vi "pco.camera_SaveImages_Example.vi"() -> ()   [LabVIEW 2019]
uses:
  pco.camera/Camera.lvclass
  pco.recorder/Recorder.lvlib
  <vilib>/picture/picture.llb/Draw 8-Bit Pixmap.vi
  <vilib>/picture/picture.llb/Draw True-Color Pixmap.vi
panel:
  out "colormap(U8)":u32[](array[numeric])
  out "Image(U16)":u16[][](graph)
  in  "Zoom [%]":i32(c297)=26
  out "Image":picture
  out "rawImage":u16[][](array[numeric])
  in  "data_format":T1(ring)=enum."Mono16"
  in  "Image Index":u32 max=9
  in  "saveImages":bool
  in  "SavePath":path
  out "Recorded Images":u32
  in  "Quit":bool
  in  "roiY1":u64=2 min=2 max=5120 step=1
  in  "roiX1":u64=2 min=2 max=5120 step=1
  in  "roiY0":u64=1 min=1 max=5119 step=1
  in  "roiX0":u64=1 min=1 max=5119 step=1
  out "Image Height":u16
  out "Image Width":u16
  in  "dwImgCount":u32=10 caption="Required Number of Images" max=4023
  out "Error":errorcluster {"code" format="%x"}
  # "This example shows how to record an image sequence and save all images to files (and an .avi) afterwards.\nIt is a good starting point for writing own applications with file saving\nBut it will not be fail save, i.e. doesnt react on errors, just handles them forward to the end\n\nUsage:\nSelect your required image count you want to record before you start the program.\nOnce started, the camera class will be initialized and images will be recorded automatically.\nWhen acquisition has finished you can read the images by index, crop them using the ROI parameters and select a file path.\nBy clicking save, the images are saved with the selected file format using the current active roi setting.\nThis also finishes the program and will force an exit of the camera class"
  # "pco.labview"
  # "Camera Setup"
  # "Recording Control"
  # "Parameters for image readout"
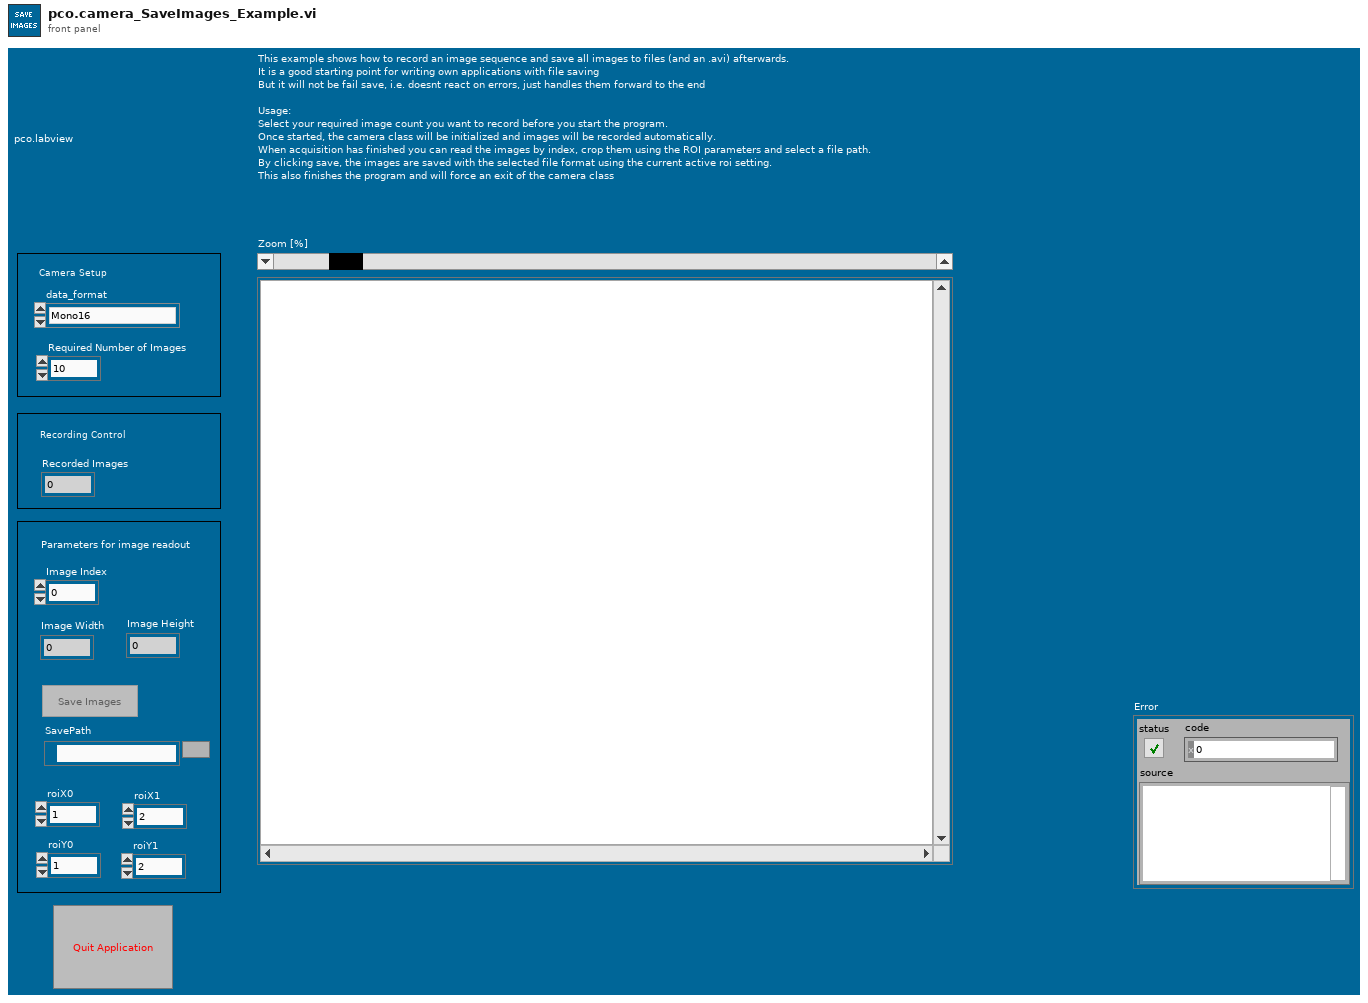
[diagram p1: front panel]
types:
  T1 = enum16{"Undefined", "Mono8", "Mono16", "BGRA8", "RGBA8", "BGRA16", "RGBA16", "CompressedMono8"}
  T2 = enum8{"Enabled", "Disabled", "Disabled and Grayed Out"}
  T3 = enum16{"sequence", "sequence non blocking", "ring buffer", "fifo", "sequence_dpcore", "sequence_non_blocking_dpcore", "ring_buffer_dpcore", "fifo_dpcore", "tif", "multitif", "pcoraw", "b16", "dicom", "multidicom"}
  T4 = typedef "Camera.lvclass/binning.ctl" = cluster{"vert":u16, "horz":u16}
  T5 = cluster{"exposure_time_s":dbl, "delay_time_s":dbl, "roi":cluster{"x0":u64, "y0":u64, "x1":u64, "y1":u64}, "timestamp_mode":u16, "pixelrate":u32, "trigger_mode":u16, "acquire_mode":u16, "metadata_mode":u16, "noisefilter_mode":u16, "binning":T4}
  T6 = cluster{"wVersion":u16, "dwIMAGE_COUNTER":u32, "dwIMAGE_TIME_US":u32, "lvTimestamp":timestamp, "bIMAGE_TIME_STATUS":u8, "wEXPOSURE_TIME_BASE":u16, "dwEXPOSURE_TIME":u32, "dwFRAMERATE_MILLIHZ":u32, "sSENSOR_TEMPERATURE":i16, "wIMAGE_SIZE_X":u16, "wIMAGE_SIZE_Y":u16, "bBINNING_X":u8, "bBINNING_Y":u8, "dwSENSOR_READOUT_FREQUENCY":u32, "wSENSOR_CONV_FACTOR":u16, "dwCAMERA_SERIAL_NO":u32, "wCAMERA_TYPE":u16, "bBIT_RESOLUTION":u8, "bSYNC_STATUS":u8, "wDARK_OFFSET":u16, "bTRIGGER_MODE":u8, "bDOUBLE_IMAGE_MODE":u8, "bCAMERA_SYNC_MODE":u8, "bIMAGE_TYPE":u8, "wCOLOR_PATTERN":u16, "wCAMERA_SUBTYPE":u16, "dwEVENT_NUMBER":u32, "wIMAGE_SIZE_X_Offset":u16, "wIMAGE_SIZE_Y_Offset":u16}[]
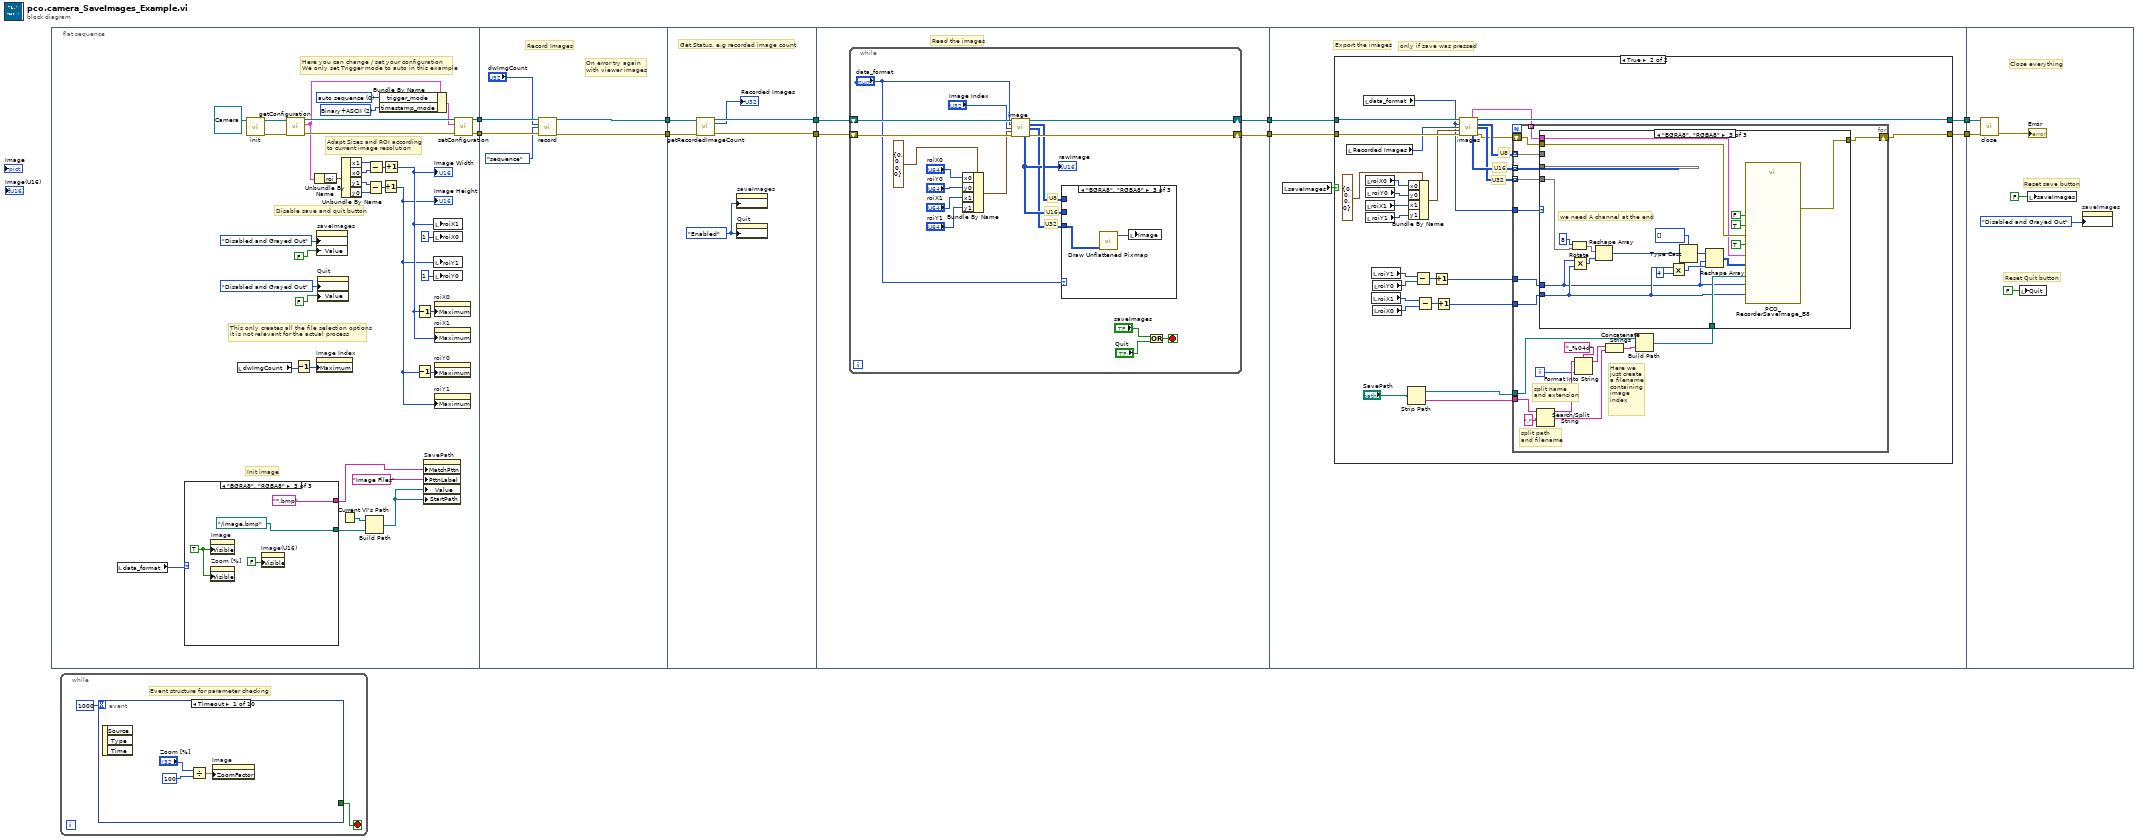
[diagram p0: block diagram]
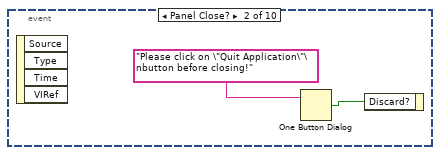
[diagram p2: hidden frame]
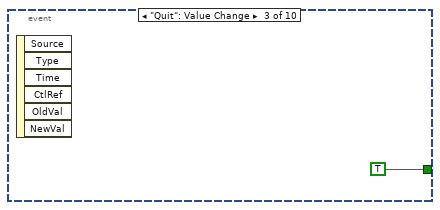
[diagram p3: hidden frame]
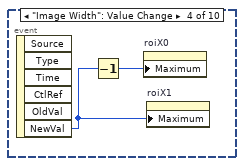
[diagram p4: hidden frame]
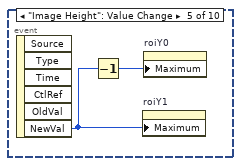
[diagram p5: hidden frame]
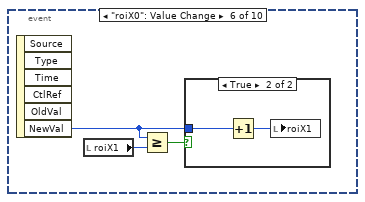
[diagram p6: hidden frame]
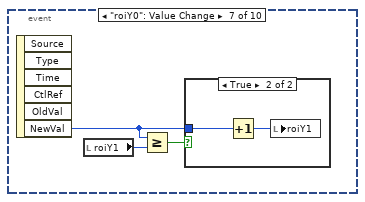
[diagram p8: hidden frame]
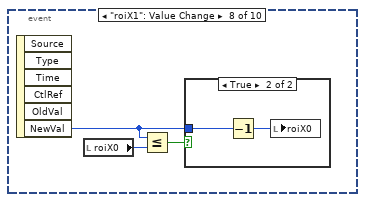
[diagram p10: hidden frame]
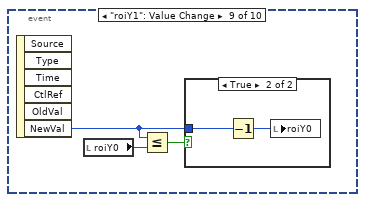
[diagram p12: hidden frame]
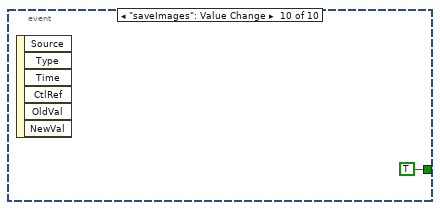
[diagram p14: hidden frame]
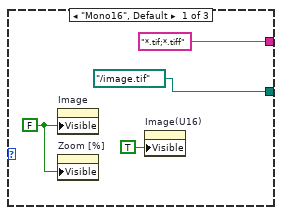
[diagram p15: hidden frame]
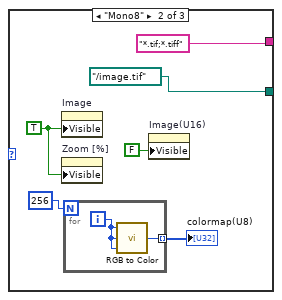
[diagram p16: hidden frame]
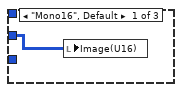
[diagram p17: hidden frame]
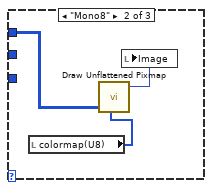
[diagram p18: hidden frame]
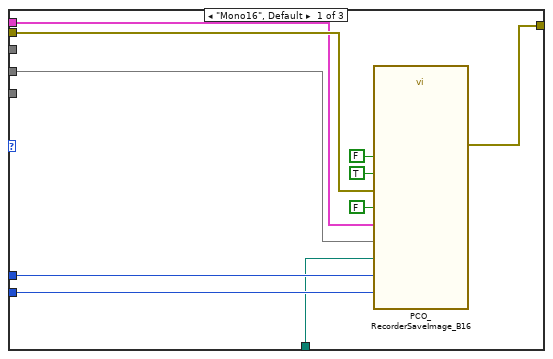
[diagram p20: hidden frame]
diagram:
  n1 = flat-sequence {
    tunnel: [w37] -> w10
    tunnel: [w36] -> w9
    tunnel: w10 -> [w68]
    tunnel: w9 -> [w67]
    tunnel: [w65] -> w8
    tunnel: [w64] -> w7
    tunnel: w8 -> [w74]
    tunnel: w7 -> [w73]
    tunnel: [w72] -> w6
    tunnel: [w71] -> w5
    tunnel: w6 -> [w77]
    tunnel: w5 -> [w78]
    tunnel: [w76] -> w4
    tunnel: [w75] -> w2
    tunnel: w4 -> [w106]
    tunnel: [w105] -> w3
    tunnel: w2 -> [w104]
    tunnel: [w103] -> w1
    tunnel: w3 -> [w201]
    tunnel: w1 -> [w200]
    frame #0 {
      w21 = u16 2 items=["OFF", "Binary", "Binary+ASCII", "ASCII"] ("TimestampMode")
      w43 = u16 0 items=["auto sequence"=0, "software trigger"=1, "external exposure start & software trigger"=2, "external exposure control"=3, "external synchronized"=4, "fast external exposure control"=5, "external CDS control"=6, "slow external exposure control"=7, "external synchronized HDSDI"=258] ("TriggerMode")
      # "Init image"
      # "This only creates all the file selection options\nit is not relevant for the actual process"
      # "Adapt Sizes and ROI according\nto current image resolution"
      # "Disable save and quit button"
      # "Here you can change / set your configuration\nWe only set Trigger mode to auto in this example"
      n2 = local read "data_format"() -> (w13:T1)
      n3 = case shown="\"BGRA8\", \"RGBA8\"" w13 {
        tunnel: [path "../image.tif" ("SavePath") path "../image.tif" ("SavePath") path "../image.bmp" ("SavePath")] -> w12
        tunnel: ["*.tif;*.tiff" ("pattern (all files)") "*.tif;*.tiff" ("pattern (all files)") "*.bmp" ("pattern (all files)")] -> w11
        frame "Mono16", Default {
          w49 = FALSE ("Visible")
          n4 = property on="Image" class="Pict"("Visible"=w49) -> ()  [unwired: 2 in, 2 out]
          n5 = property on="Zoom [%]" class="Scroll (strict)"("Visible"=w49) -> ()  [unwired: 2 in, 2 out]
          n6 = property on="Image(U16)" class="IntGraph (strict)"("Visible"=TRUE) -> ()  [unwired: 2 in, 2 out]
        }
        frame "Mono8" {
          w55 = TRUE ("Visible")
          n7 = property on="Image" class="Pict"("Visible"=w55) -> ()  [unwired: 2 in, 2 out]
          n8 = property on="Zoom [%]" class="Scroll (strict)"("Visible"=w55) -> ()  [unwired: 2 in, 2 out]
          n9 = for {
            N: 256 -> [_]
            tunnel: [w57] -> w54 mode=indexing
            i -> [w58]
            n10 = call <vilib>:"RGB to Color.vi"("B"=w58, "G"=w58, "R"=w58) -> ("Color"=w57:u32)
          }
          "colormap(U8)" <- w54
          n11 = property on="Image(U16)" class="IntGraph (strict)"("Visible"=FALSE) -> ()  [unwired: 2 in, 2 out]
        }
        frame "BGRA8", "RGBA8" {
          w61 = TRUE ("Visible")
          n12 = property on="Image" class="Pict"("Visible"=w61) -> ()  [unwired: 2 in, 2 out]
          n13 = property on="Zoom [%]" class="Scroll (strict)"("Visible"=w61) -> ()  [unwired: 2 in, 2 out]
          n14 = property on="Image(U16)" class="IntGraph (strict)"("Visible"=FALSE) -> ()  [unwired: 2 in, 2 out]
        }
      }
      n15 = local read "dwImgCount"() -> (w14:u32)
      n16 = call-dynamic "init.vi"("Camera in"=refnum<class "Camera.lvclass"> refnum ("PCOCamera in")) -> ("Camera out"=w45:refnum<class "Camera.lvclass">, "error out"=w44:errorcluster)  [unwired: 8 in]
      n17 = call-dynamic "getConfiguration.vi"("error in (no error)"=w44, "Camera in"=w45) -> ("error out"=w41:errorcluster, "configuration"=w31:T5, "Camera out"=w42:refnum<class "Camera.lvclass">)  [unwired: 7 in]
      n18 = Decrement(x=w14) -> (x-1=w15:u32)
      n19 = Unbundle By Name(w31) -> ("roi"=w30:cluster{"x0":u64, "y0":u64, "x1":u64, "y1":u64})
      n20 = property on="Image Index" class="DigNum (strict)"("Maximum"=w15) -> ()  [unwired: 2 in, 2 out]
      n21 = property on="saveImages" class="Bool (strict)"("DisabledEnum"=T2."Disabled and Grayed Out" ("Disabled"), "Value"=FALSE ("Stop")) -> ()  [unwired: 2 in, 2 out]
      n22 = property on="Quit" class="Bool (strict)"("DisabledEnum"=T2."Disabled and Grayed Out" ("Disabled"), "Value"=FALSE ("Stop")) -> ()  [unwired: 2 in, 2 out]
      n23 = Current VI's Path() -> (path=w18:path)
      n24 = Unbundle By Name(w30) -> ("x1"=w28:u64, "x0"=w29:u64, "y1"=w26:u64, "y0"=w27:u64)
      n25 = Build Path(base path=w18, name or relative path=w12) -> (appended path=w16:path)
      n26 = Subtract(x=w26, y=w27) -> (x-y=w24:u64)
      n27 = Subtract(x=w28, y=w29) -> (x-y=w25:u64)
      n28 = Bundle By Name(cluster=w31, "trigger_mode"=w43, "timestamp_mode"=w21) -> (w40:T5)
      n29 = Increment(x=w24) -> (x+1=w22:u64)
      "Image Height" <- w22
      n30 = Increment(x=w25) -> (x+1=w23:u64)
      "Image Width" <- w23
      n31 = Decrement(x=w23) -> (x-1=w33:u64)
      n32 = Decrement(x=w22) -> (x-1=w32:u64)
      n33 = property on="SavePath" class="Path"("MatchPttn"=w11, "PttnLabel"="Image Files" ("pattern label"), "Value"=w16, "StartPath"=w16) -> ()  [unwired: 2 in, 2 out]
      n34 = local write "roiX1"(w23) -> ()
      n35 = local write "roiX0"(u16 1 ("roiY0")) -> ()
      n36 = local write "roiY1"(w22) -> ()
      n37 = local write "roiY0"(u16 1 ("roiY0")) -> ()
      n38 = property on="roiX0" class="DigNum (strict)"("Maximum"=w33) -> ()  [unwired: 2 in, 2 out]
      n39 = property on="roiX1" class="DigNum (strict)"("Maximum"=w23) -> ()  [unwired: 2 in, 2 out]
      n40 = property on="roiY0" class="DigNum (strict)"("Maximum"=w32) -> ()  [unwired: 2 in, 2 out]
      n41 = property on="roiY1" class="DigNum (strict)"("Maximum"=w22) -> ()  [unwired: 2 in, 2 out]
      n42 = call-dynamic "setConfiguration.vi"("error in (no error)"=w41, "configuration"=w40, "Camera in"=w42) -> ("error out"=w36:errorcluster, "Camera out"=w37:refnum<class "Camera.lvclass">)  [unwired: 7 in]
    }
    frame #1 {
      # "On error try again \nwith viewer images"
      # "Record Images"
      n43 = call-dynamic "record.vi"("Camera in"=w68, "num_images"="dwImgCount", "record_mode"=T3."sequence", "error in (no error)"=w67) -> ("Camera out"=w65:refnum<class "Camera.lvclass">, "error out"=w64:errorcluster)  [unwired: 10 in]
    }
    frame #2 {
      w69 = T2."Enabled" ("Disabled")
      # "Get Status, e.g recorded image count"
      n44 = call-dynamic "getRecordedImageCount.vi"("Camera in"=w74, "error in (no error)"=w73) -> ("Camera out"=w72:refnum<class "Camera.lvclass">, "recorded_image_count"=→"Recorded Images":u32, "error out"=w71:errorcluster)  [unwired: 11 in]
      n45 = property on="saveImages" class="Bool (strict)"("DisabledEnum"=w69) -> ()  [unwired: 2 in, 2 out]
      n46 = property on="Quit" class="Bool (strict)"("DisabledEnum"=w69) -> ()  [unwired: 2 in, 2 out]
    }
    frame #3 {
      # "Read the images"
      n47 = while {
        shift-right: [w94] -> w76
        shift-left: w77 -> [w96]
        shift-right: [w89] -> w75
        shift-left: w78 -> [w95]
        stop <- w87 stop-if-true
        # "U32"
        # "U16"
        # "U8"
        n48 = Bundle By Name(cluster=cluster{"x0":u64, "y0":u64, "x1":u64, "y1":u64} {"x0"=0, "y0"=0, "x1"=0, "y1"=0} ("roi"), "x0"="roiX0", "y0"="roiY0", "x1"="roiX1", "y1"="roiY1") -> (w85:cluster{"x0":u64, "y0":u64, "x1":u64, "y1":u64})
        n49 = call-dynamic "image.vi"("Camera in"=w96, "data_format"="data_format", "image_index"="Image Index", "roi"=w85, "error in (no error)"=w95) -> ("Camera out"=w94:refnum<class "Camera.lvclass">, "image (U8)"=w82:u8[][], "image (U32)"=w80:u32[][], "raw_image (U16)"=w81:u16[][], "error out"=w89:errorcluster)  [unwired: 3 in, 3 out]
        "rawImage" <- w81
        n50 = case shown="\"BGRA8\", \"RGBA8\"" "data_format" {
          tunnel: w80 -> [_ _ w102]
          tunnel: w82 -> [_ w100 _]
          tunnel: w81 -> [w97 _ _]
          frame "Mono16", Default {
            n51 = local write "Image(U16)"(w97) -> ()
          }
          frame "Mono8" {
            n52 = local read "colormap(U8)"() -> (w99:u32[])
            n53 = call-poly <vilib>:"Draw Unflattened Pixmap.vi"("data"=w100, "color table"=w99) -> ("new picture"=w98:picture)  [unwired: 7 in]
            n54 = local write "Image"(w98) -> ()
          }
          frame "BGRA8", "RGBA8" {
            n55 = call-poly <vilib>:"Draw Unflattened Pixmap.vi"("data (RGB format)"=w102) -> ("new picture"=w101:picture)  [unwired: 8 in]
            n56 = local write "Image"(w101) -> ()
          }
        }
        n57 = Or(x="saveImages", y="Quit") -> (x .or. y?=w87:bool)
      }
    }
    frame #4 {
      # "only if save was pressed"
      # "Export the images"
      n58 = local read "saveImages"() -> (w107:bool)
      n59 = case shown="True" w107 {
        tunnel: w106 -> [w109 w136]
        tunnel: [w109 w125] -> w105
        tunnel: w104 -> [w108 w137]
        tunnel: [w108 w119] -> w103
        frame False {
        }
        frame True {
          # "U32"
          # "U16"
          # "U8"
          n60 = local read "Recorded Images"() -> (w129:u32)
          n61 = local read "data_format"() -> (w124:T1)
          n62 = local read "roiX0"() -> (w134:u64)
          n63 = local read "roiX1"() -> (w132:u64)
          n64 = local read "roiY0"() -> (w133:u64)
          n65 = local read "roiY1"() -> (w131:u64)
          n66 = local read "roiY1"() -> (w116:u64)
          n67 = local read "roiX1"() -> (w114:u64)
          n68 = local read "roiY0"() -> (w115:u64)
          n69 = local read "roiX0"() -> (w113:u64)
          n70 = Strip Path(path="SavePath") -> (stripped path=w121:path, name=w122:string)
          n71 = Bundle By Name(cluster=cluster{"x0":u64, "y0":u64, "x1":u64, "y1":u64} {"x0"=0, "y0"=0, "x1"=0, "y1"=0} ("roi"), "x0"=w134, "y0"=w133, "x1"=w132, "y1"=w131) -> (w130:cluster{"x0":u64, "y0":u64, "x1":u64, "y1":u64})
          n72 = Subtract(x=w116, y=w115) -> (x-y=w118:u64)
          n73 = Subtract(x=w114, y=w113) -> (x-y=w117:u64)
          n74 = Increment(x=w118) -> (x+1=w111:u64)
          n75 = Increment(x=w117) -> (x+1=w112:u64)
          n76 = call-dynamic "images.vi"("Camera in"=w136, "data_format"=w124, "image_count"=w129, "roi"=w130, "error in (no error)"=w137) -> ("meta_data_list"=w110:T6, "Camera out"=w125:refnum<class "Camera.lvclass">, "image_list (U8)"=w128:u8[][][], "image_list (U32)"=w126:u32[][][], "raw_image_list (U16)"=w127:u16[][][], "error out"=w120:errorcluster)  [unwired: 3 in, 2 out]
          n77 = for {
            tunnel: w128 -> [w156] mode=indexing
            tunnel: w127 -> [w155] mode=indexing
            tunnel: w126 -> [w139] mode=indexing
            tunnel: w124 -> [w147]
            tunnel: w122 -> [w146]
            tunnel: w121 -> [w145]
            shift-right: [w143] -> w119
            shift-left: w120 -> [w144]
            tunnel: w112 -> [w140]
            tunnel: w111 -> [w141]
            tunnel: w110 -> [w142] mode=indexing
            i -> [w148]
            # "Here we \njust create\na filename\ncontaining\nimage \nindex"
            # "split path \nand filename"
            # "split name \nand extension"
            n78 = Search/Split String(string=w146, search string/char (-)=".") -> (substring before match=w152:string, match + rest of string=w153:string)  [unwired: 1 in, 1 out]
            n79 = Format Into String(format string="_%04d", initial string=w152, w148) -> (resulting string=w154:string)  [unwired: 1 in, 1 out]
            n80 = Concatenate Strings(w154, w153) -> (w149:string)
            n81 = Build Path(base path=w145, name or relative path=w149) -> (appended path=w138:path)
            n82 = case shown="\"BGRA8\", \"RGBA8\"" w147 {
              tunnel: w156 -> [_ w173 _]
              tunnel: w155 -> [w161 _ _]
              tunnel: w141 -> [w163 w171 w180]
              tunnel: w140 -> [w162 w170 w181]
              tunnel: w144 -> [w160 w172 w192]
              tunnel: [w159 w169 w191] -> w143
              tunnel: w142 -> [w158 w168 w190]
              tunnel: w139 -> [_ _ w178]
              tunnel: w138 -> [w157 w167 w189]
              frame "Mono16", Default {
                n83 = call "PCO_RecorderSaveImage_B16.vi"("pImgBuf"=w161, "wWidth"=w162, "wHeight"=w163, "szFilePath"=w157, "error in (no error)"=w160, "isColor"=FALSE, "bIsBitmap"=FALSE, "PCO_METADATA_STRUCT"=w158, "bOverwrite"=TRUE) -> ("error out"=w159:errorcluster)  [unwired: 9 in, 1 out]
              }
              frame "Mono8" {
                n84 = call "PCO_RecorderSaveImage_B8.vi"("pImgBuf"=w173, "wWidth"=w170, "wHeight"=w171, "szFilePath"=w167, "error in (no error)"=w172, "isColor"=FALSE, "bIsBitmap"=FALSE, "PCO_METADATA_STRUCT"=w168, "bOverwrite"=TRUE) -> ("error out"=w169:errorcluster)  [unwired: 9 in, 1 out]
              }
              frame "BGRA8", "RGBA8" {
                # "we need A channel at the end"
                n85 = Rotate(1:w178, 2:i16 8 ("y")) -> (0:w177:u32[][])
                n86 = Multiply(x=w180, y=w181) -> (x*y=w183:u64)
                n87 = Reshape Array(w177, w183) -> (w182:u32[])
                n88 = Multiply(x=w181, y=u64 4) -> (x*y=w187:u64)
                n89 = Type Cast(type=u8[] [] ("image_list (U32)"), x=w182) -> (*(type *) &x=w188:u8[])
                n90 = Reshape Array(w188, w180, w187) -> (w184:u8[][])
                n91 = call "PCO_RecorderSaveImage_B8.vi"("pImgBuf"=w184, "wWidth"=w181, "wHeight"=w180, "szFilePath"=w189, "error in (no error)"=w192, "isColor"=TRUE, "bIsBitmap"=FALSE, "PCO_METADATA_STRUCT"=w190, "bOverwrite"=TRUE) -> ("error out"=w191:errorcluster)  [unwired: 9 in, 1 out]
              }
            }
          }
        }
      }
    }
    frame #5 {
      # "Reset Quit button"
      # "Close everything"
      # "Reset save button"
      n92 = call-dynamic "close.vi"("error in (no error)"=w200, "Camera in"=w201) -> ("error out"=→"Error":errorcluster)  [unwired: 9 in]
      n93 = local write "Quit"(FALSE ("Stop")) -> ()
      n94 = local write "saveImages"(FALSE ("Stop")) -> ()
      n95 = property on="saveImages" class="Bool (strict)"("DisabledEnum"=T2."Disabled and Grayed Out" ("Disabled")) -> ()  [unwired: 2 in, 2 out]
    }
  }
  n96 = while {
    stop <- w202 stop-if-true
    # "Event structure for parameter checking"
    n97 = event shown="[0] Timeout" {
      selector: _ -> [_ _ _ _ _ _ _ _ _ _]
      dyn-events: _ -> [_ _ _ _ _ _ _ _ _ _]
      timeout: 1000 -> [_ _ _ _ _ _ _ _ _ _]
      tunnel: [_ _ TRUE _ _ _ _ _ _ TRUE] -> w202
      event Timeout {
        n98 = event-data() -> ()  [unwired: 1 in, 3 out]
        n99 = Divide(x="Zoom [%]", y=100 ("Zoom [%]")) -> (x/y=w206:dbl)
        n100 = property on="Image" class="Pict"("ZoomFactor"=w206) -> ()  [unwired: 2 in, 2 out]
      }
      event Panel Close? {
        n101 = event-data() -> ()  [unwired: 1 in, 4 out]
        n102 = One Button Dialog(message="Please click on \"Quit Application\"\nbutton before closing!") -> (true=w207:bool)  [unwired: 1 in]
        n103 = event-data("Discard?"=w207) -> ()  [unwired: 1 in, 1 out]
      }
      event "Quit": Value Change {
        n104 = event-data() -> ()  [unwired: 1 in, 6 out]
      }
      event "Image Width": Value Change {
        n105 = event-data() -> ("NewVal"=w210:u16)  [unwired: 1 in, 5 out]
        n106 = Decrement(x=w210) -> (x-1=w211:u16)
        n107 = property on="roiX0" class="DigNum (strict)"("Maximum"=w211) -> ()  [unwired: 2 in, 2 out]
        n108 = property on="roiX1" class="DigNum (strict)"("Maximum"=w210) -> ()  [unwired: 2 in, 2 out]
      }
      event "Image Height": Value Change {
        n109 = event-data() -> ("NewVal"=w212:u16)  [unwired: 1 in, 5 out]
        n110 = Decrement(x=w212) -> (x-1=w213:u16)
        n111 = property on="roiY1" class="DigNum (strict)"("Maximum"=w212) -> ()  [unwired: 2 in, 2 out]
        n112 = property on="roiY0" class="DigNum (strict)"("Maximum"=w213) -> ()  [unwired: 2 in, 2 out]
      }
      event "roiX0": Value Change {
        n113 = event-data() -> ("NewVal"=w214:u64)  [unwired: 1 in, 5 out]
        n114 = local read "roiX1"() -> (w216:u64)
        n115 = Greater Or Equal?(x=w214, y=w216) -> (x >= y?=w215:bool)
        n116 = case shown="True" w215 {
          tunnel: w214 -> [_ w218]
          frame False {
          }
          frame True {
            n117 = Increment(x=w218) -> (x+1=w217:u64)
            n118 = local write "roiX1"(w217) -> ()
          }
        }
      }
      event "roiY0": Value Change {
        n119 = event-data() -> ("NewVal"=w219:u64)  [unwired: 1 in, 5 out]
        n120 = local read "roiY1"() -> (w221:u64)
        n121 = Greater Or Equal?(x=w219, y=w221) -> (x >= y?=w220:bool)
        n122 = case shown="True" w220 {
          tunnel: w219 -> [_ w223]
          frame False {
          }
          frame True {
            n123 = Increment(x=w223) -> (x+1=w222:u64)
            n124 = local write "roiY1"(w222) -> ()
          }
        }
      }
      event "roiX1": Value Change {
        n125 = event-data() -> ("NewVal"=w224:u64)  [unwired: 1 in, 5 out]
        n126 = local read "roiX0"() -> (w226:u64)
        n127 = Less Or Equal?(x=w224, y=w226) -> (x <= y?=w225:bool)
        n128 = case shown="True" w225 {
          tunnel: w224 -> [_ w228]
          frame False {
          }
          frame True {
            n129 = Decrement(x=w228) -> (x-1=w227:u64)
            n130 = local write "roiX0"(w227) -> ()
          }
        }
      }
      event "roiY1": Value Change {
        n131 = event-data() -> ("NewVal"=w229:u64)  [unwired: 1 in, 5 out]
        n132 = local read "roiY0"() -> (w231:u64)
        n133 = Less Or Equal?(x=w229, y=w231) -> (x <= y?=w230:bool)
        n134 = case shown="True" w230 {
          tunnel: w229 -> [_ w233]
          frame False {
          }
          frame True {
            n135 = Decrement(x=w233) -> (x-1=w232:u64)
            n136 = local write "roiY0"(w232) -> ()
          }
        }
      }
      event "saveImages": Value Change {
        n137 = event-data() -> ()  [unwired: 1 in, 6 out]
      }
    }
  }
